vi "Register Event.vi"   [LabVIEW 2019, in "FootScan Engine Event.lvlib"]
uses:
  FootScan Engine Event.lvlib
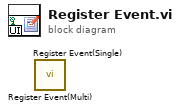
[diagram p0: block diagram]
diagram:
  n1 = call "Register Event(Multi).vi"() -> ()  [unwired: 11 in, 1 out]
  n2 = call "Register Event(Single).vi"() -> ()  [unwired: 11 in, 1 out]
